vi "Voltage Measurement.vi"() -> ()   [LabVIEW 2021, in "Main.lvlib"]
uses:
  Main.lvlib
  <instrlib>/niDMM/nidmm.llb/niDMM Resolution in Digits.ctl
  SMU/SMU.lvlib
  DMM/DMM.lvlib
panel:
  out "Signal Out of Range":bool
  out "Measurement":dbl format="%.6p"
  in  "Resolution in Digits":T1=5.5 items=["3 1/2"=3.5, "4 1/2"=4.5, "5 1/2"=5.5, "6 1/2"=6.5, "7 1/2"=7.5]
  in  "Range":dbl=10.0 format="%.2f"
  in  "Device Name":refnum<k15>="Dev1"
  out "error out":errorcluster
  out "Current Measurement":dbl
  out "Voltage Measurement":dbl
  in  "error in":errorcluster
  in  "Voltage Level Range":dbl=6.0 format="%.5p"
  in  "Voltage Level":dbl=2.0 format="%.5p"
  in  "Vin SMU Channel":string="0"
  in  "Current Limit Range":dbl=0.01 format="%.3p"
  in  "Current Limit":dbl=0.01 format="%.3p"
  in  "Vin SMU":refnum<k15>="Dev1"
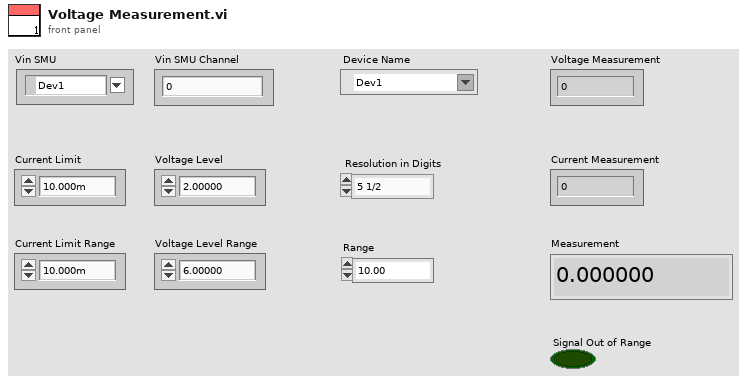
[diagram p1: front panel]
types:
  T1 = typedef "niDMM Resolution in Digits.ctl" = dbl
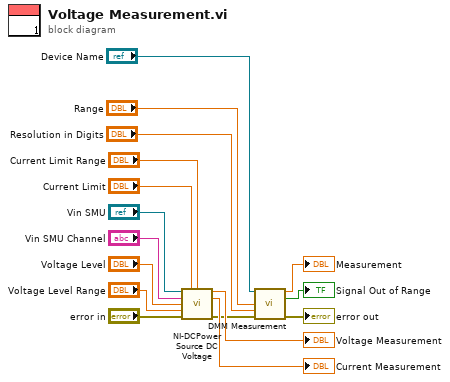
[diagram p0: block diagram]
diagram:
  n1 = call "NI-DCPower Source DC Voltage.vi"("Vin SMU"="Vin SMU", "Current Limit"="Current Limit", "Current Limit Range"="Current Limit Range", "Vin SMU Channel"="Vin SMU Channel", "Voltage Level"="Voltage Level", "Voltage Level Range"="Voltage Level Range", "error in"="error in") -> ("Voltage Measurement"=→"Voltage Measurement":dbl, "Current Measurement"=→"Current Measurement":dbl, "error out"=w6:errorcluster)  [unwired: 6 in]
  n2 = call "DMM Measurement.vi"("Device Name"="Device Name", "Range"="Range", "Resolution in Digits"="Resolution in Digits", "error in"=w6) -> ("Measurement"=→"Measurement":dbl, "Signal Out of Range"=→"Signal Out of Range":bool, "error out"=→"error out":errorcluster)  [unwired: 9 in]
